vi "v0.2_vout_http.vi"(8 "error in (no error)":errorcluster, 10 "Vout":dbl, 11 "mbed.lvclass IN":refnum<class "mbed.lvclass">) -> (0 "error out":errorcluster, 3 "mbed.lvclass OUT":refnum<class "mbed.lvclass">)   [LabVIEW 2011]
doc: "<B>Control de Velocidad</B>\n\nCabia el voltaje a la salida del amplificador operacional. Esto controla la velocidad del servomotor cuando se lo configura en modo de Control de Velocidad\n<B>Vout</B> Un valor entre -10 y 10 V"
uses:
  C:/mbed/Transport Mechanisms/mbed/mbed.lvclass
  C:/mbed/mbed Interface/RPCFunction/RPCFunction.lvclass
panel:
  # "CAMBIA EL VOLTAJE DE SALIDA AL DRIVER"
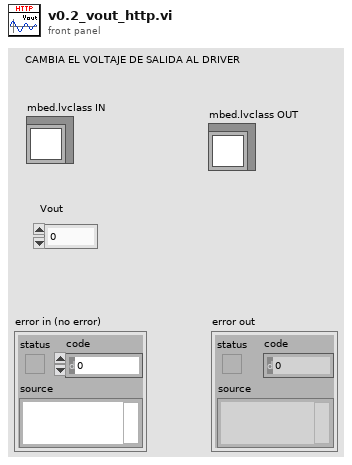
[diagram p1: front panel]
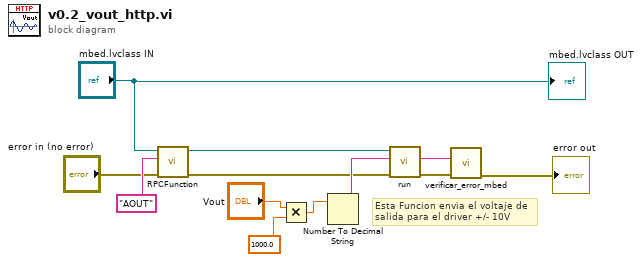
[diagram p0: block diagram]
diagram:
  # "Esta Funcion envia el voltaje de\nsalida para el driver +/- 10V"
  n1 = call "RPCFunction.vi"("error in (no error)"="error in (no error)", "Existing Obj Name"="AOUT", "mbed_LVLibrary.lvlib:mbed.lvclass"="mbed.lvclass IN") -> ("error out"=w4:errorcluster, "mbed_LVLibrary.lvlib:Packet.lvclass 2"=w11:refnum<class "RPCFunction.lvclass">)  [unwired: 6 in, 1 out]
  n2 = Multiply(x="Vout", y=1000.0) -> (x*y=w7:dbl)
  n3 = Number To Decimal String(number=w7) -> (decimal integer string=w10:string)  [unwired: 1 in]
  n4 = call "run.vi"("error in (no error)"=w4, "Input"=w10, "Packet in"=w11) -> ("error out"=w2:errorcluster, "Output"=w3:string)  [unwired: 6 in, 1 out]
  n5 = call "verificar_error_mbed.vi"("error in (no error)"=w2, "desde_mbed"=w3) -> ("error out"=→"error out":errorcluster)  [unwired: 8 in, 1 out]
  "mbed.lvclass OUT" <- "mbed.lvclass IN"
